vi "LVPortGetMatlabCorePaths.vi"() -> (3 "LibPath":path)   [LabVIEW 2017]
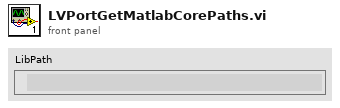
[diagram p1: front panel]
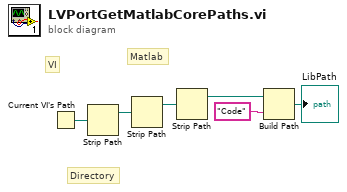
[diagram p0: block diagram]
diagram:
  # "Matlab"
  # "VI"
  # "Directory"
  n1 = Current VI's Path() -> (path=w6:path)
  n2 = Strip Path(path=w6) -> (stripped path=w5:path)  [unwired: 1 out]
  n3 = Strip Path(path=w5) -> (stripped path=w4:path)  [unwired: 1 out]
  n4 = Strip Path(path=w4) -> (stripped path=w2:path)  [unwired: 1 out]
  n5 = Build Path(base path=w2, name or relative path="Code") -> (appended path=→"LibPath":path)
